vi "TorsionDiskIO.vi"(8 "error in":errorcluster, 9 "Deflection Limit":i32=650, 10 "Motor Voltage":i16, 11 "FPGA VI Reference In":refnum<k20>) -> (0 "error out":errorcluster, 1 "Killswitch Activated":bool, 2 "Encoder Positions":i32[](array[numeric]), 3 "FPGA VI Reference Out":refnum<k20>)   [LabVIEW 2013]
uses:
  <vilib>/Utility/error.llb/Error Cluster From Error Code.vi
  <vilib>/rvi/errors/niLvFpgaAdjustHostInterfaceError.vi
  <vilib>/rvi/interface/nirviReadWriteControl/nirviReadWriteControl.xnode
  torsional-fpga-interface.lvbit
  NiFpgaLv.dll
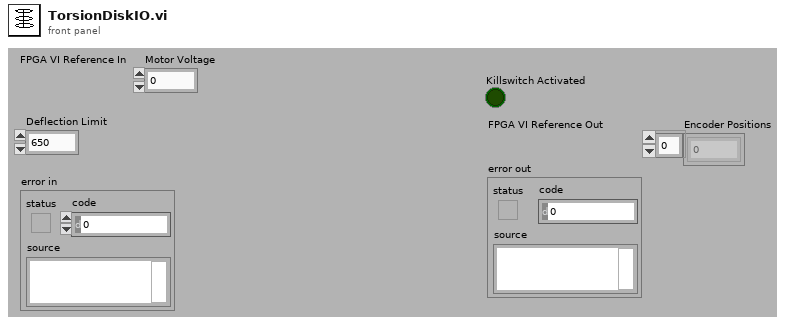
[diagram p1: front panel]
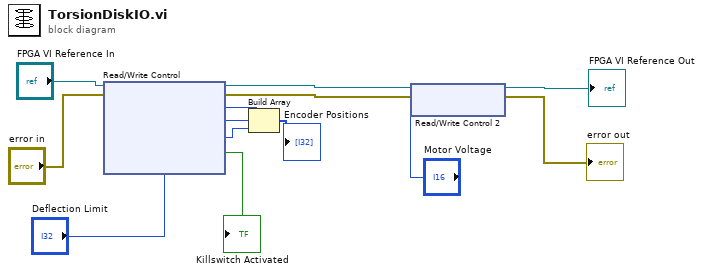
[diagram p0: block diagram]
diagram:
  n1 = xnode ("Read/Write Control")("FPGA VI Reference In"="FPGA VI Reference In", "error in"="error in", "Deflection Limit"="Deflection Limit") -> ("FPGA VI Reference Out"=w11:refnum<k20>, "error out"=w10:errorcluster, "Top Encoder"=w6:i32, "Middle Encoder"=w5:i32, "Bottom Encoder"=w4:i32, "Killswitch Activated"=→"Killswitch Activated":bool)
  n2 = Build Array(w6, w5, w4) -> (→"Encoder Positions":i32[])
  n3 = xnode ("Read/Write Control 2")("FPGA VI Reference In"=w11, "error in"=w10, "Motor Voltage"="Motor Voltage") -> ("FPGA VI Reference Out"=→"FPGA VI Reference Out":refnum<k20>, "error out"=→"error out":errorcluster)
